vi "solar_write SOLARUIRefresh.vi"(8 "error in (no error)":errorcluster, 10 "Target":string, 11 "solar in":refnum<class "solar.lvclass">) -> (0 "error out":errorcluster, 3 "solar out":refnum<class "solar.lvclass">)   [LabVIEW 2018, in "solar.lvclass"]
doc: "This refershes the Target List and window panes in the SOLAR user interface. The front panel origins are also reset to 0,0."
uses:
  solar.lvclass
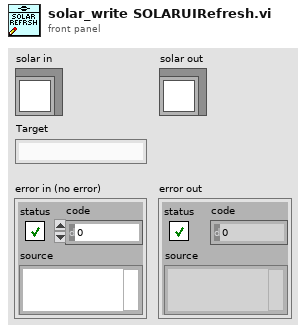
[diagram p1: front panel]
types:
  T1 = typedef "solar_ctl SOLAR Refnum.ctl" = refnum<k1>
  T2 = typedef "solar_ctl SOLAR Global.ctl" = cluster{"Targets":T3[], "AppDir":path, "solar.ini":path, "ConfigsDir":path, "CosmosDir":path, "LogsDir":path, "ExePath":path, "ExeVersion":string, "PartNum":string, "AppSetup":string, "Title":string, "Main.ini":path, "Temp.ini":path, "vSOLAR":string, "Splash.png":string, "SplashWait":i32, "SOLARUE":refnum<user-event>, "VoyagerRefnum":T4, "QTimerRefnum":T5}
  T3 = typedef "solar_ctl Target Global.ctl" = cluster{"Target":string, "Q":refnum<queue>, "UE":refnum<user-event>, "VI":refnum<vi>, "Menu":refnum<k9>, "Data":refnum<data-value>, "Attributes":variant}
  T4 = typedef "solar_voy_ctl Voyager Refnum.ctl" = refnum<k1>
  T5 = typedef "solar_qtimer_ctl Refnum.ctl" = refnum<k1>
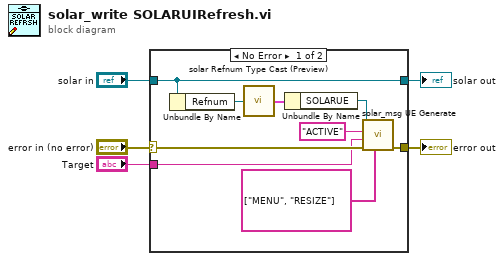
[diagram p0: block diagram]
diagram:
  n1 = case shown="No Error" "error in (no error)" {
    selector: "error in (no error)" -> [w10 w16]
    tunnel: "solar in" -> [w12 w15]
    tunnel: [w7 w16] -> w2
    tunnel: [w12 w15] -> w1
    tunnel: "Target" -> [w8 _]
    frame No Error {
      n2 = Unbundle By Name(w12) -> ("Refnum"=w14:T1)
      n3 = call "solar Refnum Type Cast (Preview).vi"("Refnum"=w14) -> ("SOLAR"=w13:T2)  [unwired: 8 in]
      n4 = Unbundle By Name(w13) -> ("SOLARUE"=w9:refnum<user-event>)
      n5 = call "solar_msg UE Generate.vi"("CMD (Array)"=string[] ["MENU", "RESIZE"], "error in (no error)"=w10, "CMD_DATA (Last)"=w8, "CMD (Last)"="ACTIVE" ("Packet"), "UserEvent in"=w9) -> ("error out"=w7:errorcluster)  [unwired: 5 in, 1 out]
    }
    frame Error {
    }
  }
  "error out" <- w2
  "solar out" <- w1
